vi "Configure Trigger (Alternation).vi"(0 "VISA resource name":refnum<visa-resource-name>, 5 "Trigger Source (0: CH1CH2)":u16(ring) items=["CH1CH2", "CH1CH3", "CH1CH4", "CH2CH3", "Ch2CH4", "CH3CH4"], 11 "error in (no error)":errorcluster) -> (4 "VISA resource name out":refnum<visa-resource-name>, 15 "error out":errorcluster)   [LabVIEW 2010, in "Agilent DSO1000 Series.lvlib"]
doc: "Configures alternation trigger settings. You specify the two channels which to trigger on by setting <B>Trigger Source</B> value."
uses:
  <instrlib>/Agilent DSO1000 Series/Agilent DSO1000 Series.lvlib
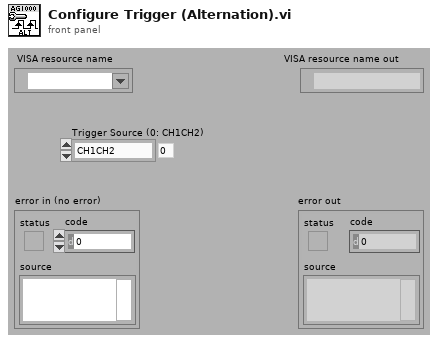
[diagram p1: front panel]
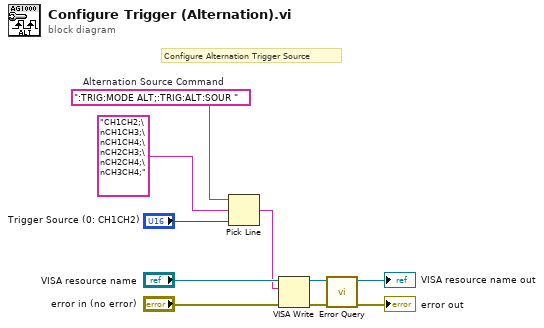
[diagram p0: block diagram]
diagram:
  w2 = ":TRIG:MODE ALT;:TRIG:ALT:SOUR "  # Alternation Source Command
  # "Configure Alternation Trigger Source"
  n1 = Pick Line(string ("")=w2, multi-line string="CH1CH2;\nCH1CH3;\nCH1CH4;\nCH2CH3;\nCH2CH4;\nCH3CH4;", line index="Trigger Source (0: CH1CH2)") -> (output string=w1:string)
  n2 = VISA Write(VISA resource name="VISA resource name", write buffer=w1, error in (no error)="error in (no error)") -> (VISA resource name out=w6:refnum<visa-resource-name>, error out=w5:errorcluster)  [unwired: 1 out]
  n3 = call <instrlib>:"Error Query.vi"("error in (no error)"=w5, "VISA resource name"=w6) -> ("error out"=→"error out":errorcluster, "VISA resource name out"=→"VISA resource name out":refnum<visa-resource-name>)  [unwired: 6 in, 2 out]
